vi "Initialize with Switch Parameters Core.vi"(8 "error in (no error)":errorcluster, 10 "Switch Parameters in":refnum<class "Abstract Switch Init Parameters.lvclass">, 11 "SLSC Switch Consumer in":refnum<class "SLSC Switch Consumer.lvclass">) -> (0 "error out":errorcluster, 3 "SLSC Switch Consumer out":refnum<class "SLSC Switch Consumer.lvclass">)   [LabVIEW 2017, in "SLSC Switch Messaging.lvlib" / "SLSC Switch Consumer.lvclass"]
uses:
  SLSC Switch Consumer.lvclass
  Includes/CDMessaging.lvlibp/Switch/Abstract Switch Init Parameters/Abstract Switch Init Parameters.lvclass
  SLSC Switch Init Parameters/SLSC Switch Init Parameters.lvclass
  C:/Users/nitest/Documents/ni/niveristand-slsc-switch-message-library/Includes/CDMessaging.lvlibp/Switch/Abstract Switch Init Parameters/Abstract Switch Init Parameters.lvclass
  SLSC Switch Consumer.lvclass/SLSC Switch Consumer.ctl
  <vilib>/SLSC_Switch/Initialize with Topology (Simulate).vi
  <vilib>/SLSC_Switch/Initialize with Topology (Override Switches).vi
  <vilib>/SLSC_Switch/SLSC Switch.lvlib
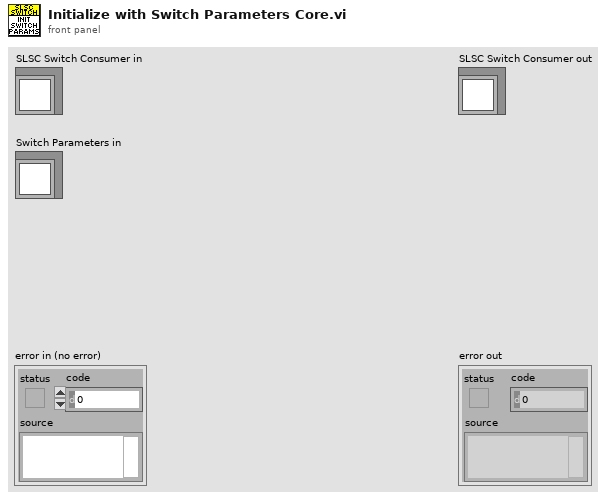
[diagram p1: front panel]
types:
  T1 = typedef "nislscslSession.ctl" = refnum<k20>
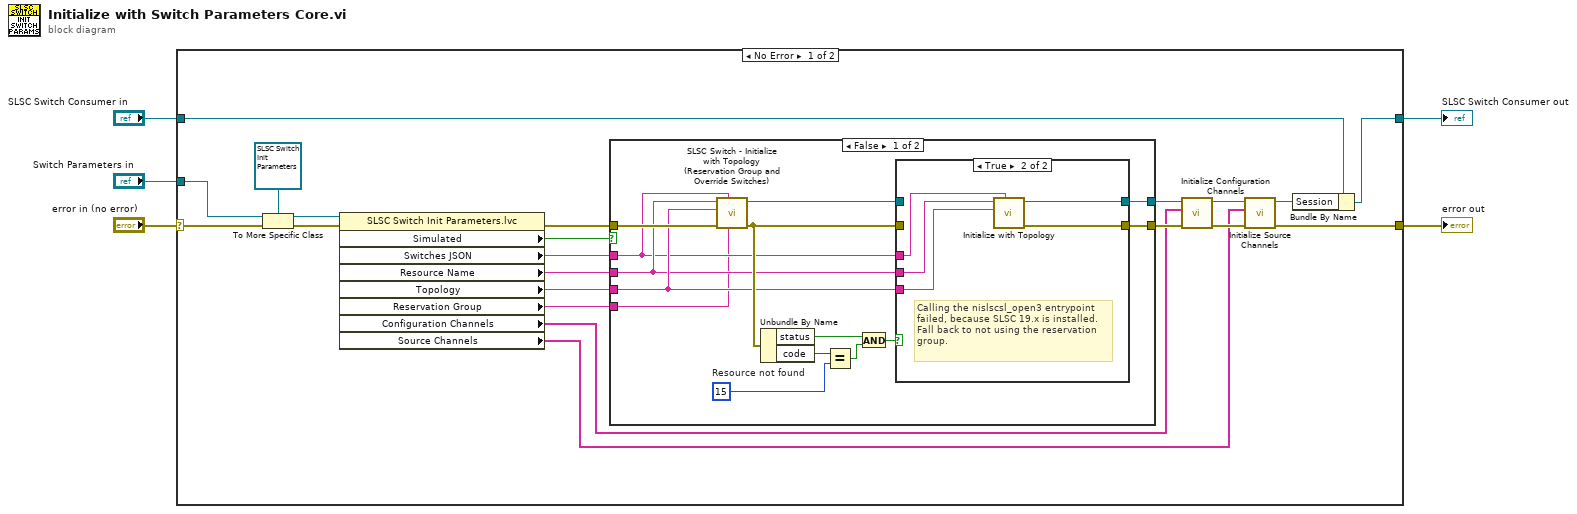
[diagram p0: block diagram]
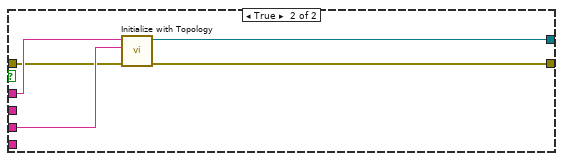
[diagram p3: hidden frame]
diagram:
  n1 = case shown="No Error" "error in (no error)" {
    selector: "error in (no error)" -> [w16 w54]
    tunnel: [w9 w54] -> w4
    tunnel: [w25 w53] -> w1
    tunnel: "SLSC Switch Consumer in" -> [w26 w53]
    tunnel: "Switch Parameters in" -> [w19 _]
    frame No Error {
      n2 = To More Specific Class(target class=refnum<class "SLSC Switch Init Parameters.lvclass"> refnum ("SLSC Switch Messaging.lvlib:SLSC Switch Init Parameters.lvclass"), reference=w19, error in=w16) -> (specific class reference=w17:refnum<class "SLSC Switch Init Parameters.lvclass">, error out=w15:errorcluster)
      n3 = property class="SLSC Switch Init Parameters.lvc"(reference=w17, error in=w15) -> (error out=w23:errorcluster, "Simulated"=w21:bool, "Switches JSON"=w24:string, "Resource Name"=w22:string, "Topology"=w20:string, "Reservation Group"=w6:string, "Configuration Channels"=w7:string[], "Source Channels"=w8:string[])  [unwired: 1 out]
      n4 = case shown="False" w21 {
        tunnel: w24 -> [w28 w50]
        tunnel: [w31 w52] -> w11
        tunnel: [w32 w51] -> w14
        tunnel: w23 -> [w40 w48]
        tunnel: w22 -> [w29 _]
        tunnel: w20 -> [w30 w49]
        tunnel: w6 -> [w27 _]
        frame False {
          w38 = 15  # Resource not found
          n5 = call "SLSC Switch - Initialize with Topology (Reservation Group and Override Switches).vi"("reservation group"=w27, "switches json"=w28, "error in (no error)"=w40, "topology"=w30, "device"=w29) -> ("error out"=w34:errorcluster, "session out"=w33:T1)  [unwired: 5 in]
          n6 = Unbundle By Name(w34) -> ("status"=w36:bool, "code"=w39:i32)
          n7 = Equal?(x=w39, y=w38) -> (x = y?=w37:bool)
          n8 = And(x=w36, y=w37) -> (x .and. y?=w35:bool)
          n9 = case shown="True" w35 {
            tunnel: w34 -> [w41 _]
            tunnel: w33 -> [w42 _]
            tunnel: [w42 w46] -> w32
            tunnel: [w41 w47] -> w31
            tunnel: w30 -> [_ w45]
            tunnel: w29 -> [_ w44]
            tunnel: w28 -> [_ w43]
            frame False {
            }
            frame True {
              # "Calling the nislscsl_open3 entrypoint\nfailed, because SLSC 19.x is installed.\nFall back to not using the reservation\ngroup."
              n10 = call-poly <vilib>:"Initialize with Topology.vi"("switches json"=w43, "topology"=w45, "device"=w44) -> ("error out"=w47:errorcluster, "session out"=w46:T1)  [unwired: 7 in]
            }
          }
        }
        frame True {
          n11 = call-poly <vilib>:"Initialize with Topology.vi"("error in (no error)"=w48, "topology"=w49, "switches json"=w50) -> ("error out"=w52:errorcluster, "session out"=w51:T1)  [unwired: 7 in]
        }
      }
      n12 = call "Initialize Configuration Channels.vi"("error in (no error)"=w11, "Configuration Channels"=w7, "Session in"=w14) -> ("error out"=w10:errorcluster, "Session out"=w13:T1)  [unwired: 7 in]
      n13 = call "Initialize Source Channels.vi"("error in (no error)"=w10, "Source Channels"=w8, "Session in"=w13) -> ("error out"=w9:errorcluster, "Session out"=w12:T1)  [unwired: 7 in]
      n14 = Bundle By Name(cluster=w26, "Session"=w12) -> (w25:refnum<class "SLSC Switch Consumer.lvclass">)
    }
    frame Error {
    }
  }
  "error out" <- w4
  "SLSC Switch Consumer out" <- w1
